vi "Build-timeline.vi"(8 "error in (no error)":errorcluster, 10 "Temp-timeline in":T1={"Previous point"={"Start time [µs]"=0, "End time [µs]"=0, "X [mm]"=0.0, "Y [mm]"=0.0, "Type"=enum."BeginJob", "Speed [mm/µs]"=0.0, "Direction [rad]"=0.0, "X [bit]"=0, "Y [bit]"=0, "Speed [bit/µs]"=0.0, "Power [W]"=0.0, "Power [bit]"=0, "JumpDelay"=0, "MarkDelay"=0, "PolyDelay"=0, "LaserOnDelay"=0, "LaserOffDelay"=0, "LaserPowerDelay"=0, "LaserEnableDelay"=0, "Xraw [mm]"=0.0, "Yraw [mm]"=0.0}, "Current point"={"Start time [µs]"=0, "End time [µs]"=0, "X [mm]"=0.0, "Y [mm]"=0.0, "Type"=enum."BeginJob", "Speed [mm/µs]"=0.0, "Direction [rad]"=0.0, "X [bit]"=0, "Y [bit]"=0, "Speed [bit/µs]"=0.0, "Power [W]"=0.0, "Power [bit]"=0, "JumpDelay"=0, "MarkDelay"=0, "PolyDelay"=0, "LaserOnDelay"=0, "LaserOffDelay"=0, "LaserPowerDelay"=0, "LaserEnableDelay"=0, "Xraw [mm]"=0.0, "Yraw [mm]"=0.0}, "Path"=[], "Current properties"={"ItemID"=0, "Start time"=0, "EffectiveOffset"=[0.0, 0.0], "EffectiveTranfsorm"=[[1.0, 0.0], [0.0, 1.0]], "Z-Offset"=0.0, "Units"=enum."mm", "LaserPower"=0, "Started"=FALSE, "Enabled"=FALSE, "FieldOffset"=[0.0, 0.0], "Offset"=[0.0, 0.0], "TransformEnable"=TRUE, "XYCalFactor"=196.0, "JumpSpeed"={"unit/us"=0.0, "Tick interval us"=0, "Bits per interval"=0}, "MarkSpeed"={"unit/us"=0.0, "Tick interval us"=0, "Bits per interval"=0}}}, 11 "JumpAbs in":refnum<class "JumpAbs.lvclass">) -> (0 "error out":errorcluster, 2 "Temp-timeline":T1={"Previous point"={"Start time [µs]"=0, "End time [µs]"=0, "X [mm]"=0.0, "Y [mm]"=0.0, "Type"=enum."BeginJob", "Speed [mm/µs]"=0.0, "Direction [rad]"=0.0, "X [bit]"=0, "Y [bit]"=0, "Speed [bit/µs]"=0.0, "Power [W]"=0.0, "Power [bit]"=0, "JumpDelay"=0, "MarkDelay"=0, "PolyDelay"=0, "LaserOnDelay"=0, "LaserOffDelay"=0, "LaserPowerDelay"=0, "LaserEnableDelay"=0, "Xraw [mm]"=0.0, "Yraw [mm]"=0.0}, "Current point"={"Start time [µs]"=0, "End time [µs]"=0, "X [mm]"=0.0, "Y [mm]"=0.0, "Type"=enum."BeginJob", "Speed [mm/µs]"=0.0, "Direction [rad]"=0.0, "X [bit]"=0, "Y [bit]"=0, "Speed [bit/µs]"=0.0, "Power [W]"=0.0, "Power [bit]"=0, "JumpDelay"=0, "MarkDelay"=0, "PolyDelay"=0, "LaserOnDelay"=0, "LaserOffDelay"=0, "LaserPowerDelay"=0, "LaserEnableDelay"=0, "Xraw [mm]"=0.0, "Yraw [mm]"=0.0}, "Path"=[], "Current properties"={"ItemID"=0, "Start time"=0, "EffectiveOffset"=[0.0, 0.0], "EffectiveTranfsorm"=[[1.0, 0.0], [0.0, 1.0]], "Z-Offset"=0.0, "Units"=enum."mm", "LaserPower"=0, "Started"=FALSE, "Enabled"=FALSE, "FieldOffset"=[0.0, 0.0], "Offset"=[0.0, 0.0], "TransformEnable"=TRUE, "XYCalFactor"=196.0, "JumpSpeed"={"unit/us"=0.0, "Tick interval us"=0, "Bits per interval"=0}, "MarkSpeed"={"unit/us"=0.0, "Tick interval us"=0, "Bits per interval"=0}}}, 3 "JumpAbs out":refnum<class "JumpAbs.lvclass">)   [LabVIEW 2013, in "HardwareCharacterization.lvlib" / "JumpAbs.lvclass"]
uses:
  JumpAbs.lvclass
  ScanParser/Path-buffer.ctl
  ScanParser/Point-buffer.ctl
  Elements.ctl
  ScanParser/Property-buffer.ctl
  ScanParser/Units.ctl
  ScanParser/Speed.ctl
  JumpAbs.lvclass/JumpAbs.ctl
  <vilib>/Analysis/baseanly.llb/A x Vector.vi
  <vilib>/Analysis/Matrix/Numeric/Conversions/Array To Matrix - RA2.vi
  <vilib>/Analysis/Matrix/NI_Matrix.lvlib
  <vilib>/Analysis/NI_AALBase.lvlib
  Element-XML.lvclass
  ScanParser/HC-ScanParser.lvclass
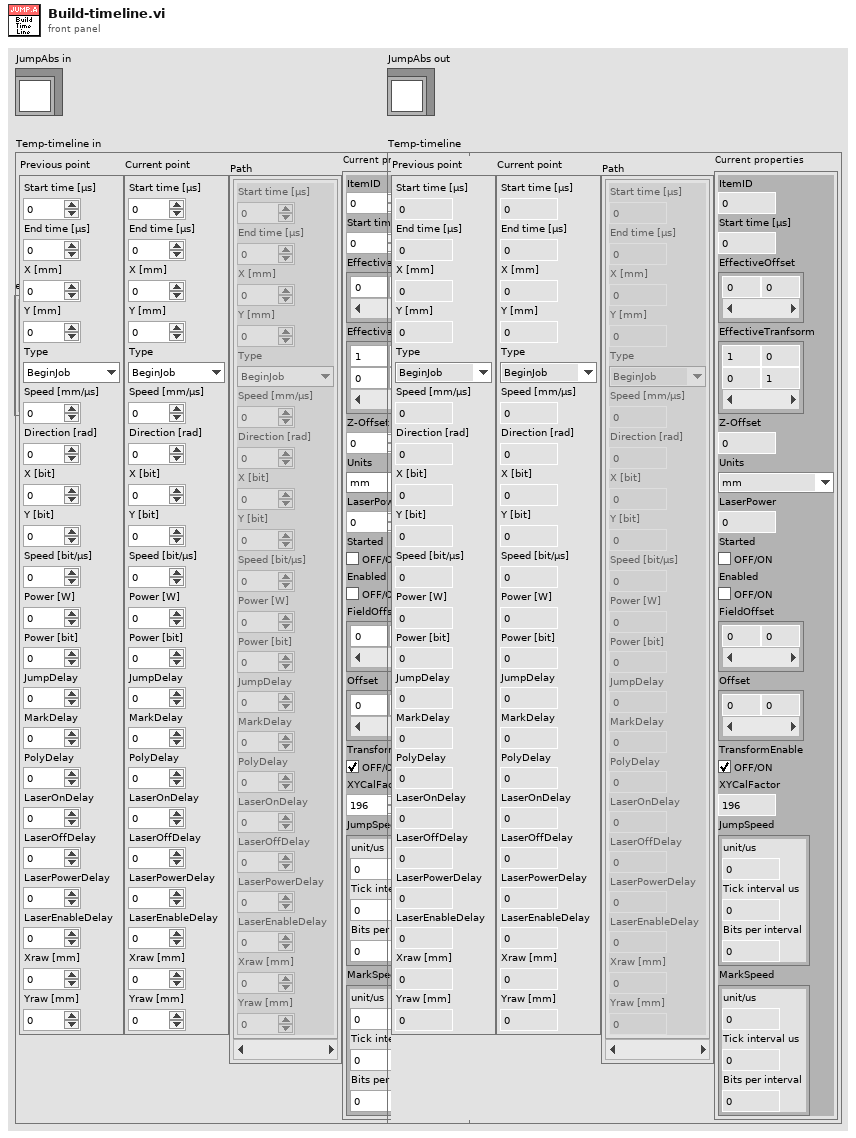
[diagram p1: front panel]
types:
  T1 = typedef "HardwareCharacterization.lvlib/HC-ScanParser.lvclass/Path-buffer.ctl" = cluster{"Previous point":T2, "Current point":T2, "Path":T2[], "Current properties":T4}
  T2 = typedef "HardwareCharacterization.lvlib/HC-ScanParser.lvclass/Point-buffer.ctl" = cluster{"Start time [µs]":i64, "End time [µs]":i64, "X [mm]":dbl, "Y [mm]":dbl, "Type":T3, "Speed [mm/µs]":dbl, "Direction [rad]":dbl, "X [bit]":i16, "Y [bit]":i16, "Speed [bit/µs]":dbl, "Power [W]":dbl, "Power [bit]":u8, "JumpDelay":i64, "MarkDelay":i64, "PolyDelay":i64, "LaserOnDelay":i64, "LaserOffDelay":i64, "LaserPowerDelay":i64, "LaserEnableDelay":i64, "Xraw [mm]":dbl, "Yraw [mm]":dbl}
  T3 = typedef "HardwareCharacterization.lvlib/Element-XML.lvclass/Elements.ctl" = enum16{"BeginJob", "WriteDigital", "WriteAnalog", "Set", "ApplicationEvent", "JumpAbs", "MarkAbs", "JumpRel", "MarkRel", "LongDelay", "EndJob"}
  T4 = typedef "HardwareCharacterization.lvlib/HC-ScanParser.lvclass/Property-buffer.ctl" = cluster{"ItemID":u32, "Start time":i64, "EffectiveOffset":dbl[], "EffectiveTranfsorm":dbl[][], "Z-Offset":sgl, "Units":T5, "LaserPower":u8, "Started":bool, "Enabled":bool, "FieldOffset":dbl[], "Offset":dbl[], "TransformEnable":bool, "XYCalFactor":dbl, "JumpSpeed":T6, "MarkSpeed":T6}
  T5 = typedef "HardwareCharacterization.lvlib/HC-ScanParser.lvclass/Units.ctl" = enum16{"bits", "mm", "inch", "mils"}
  T6 = typedef "HardwareCharacterization.lvlib/HC-ScanParser.lvclass/Speed.ctl" = cluster{"unit/us":dbl, "Tick interval us":u16, "Bits per interval":u16}
  T7 = typedef "NI_Matrix.lvlib/RealMatrix.ctl" = dbl[][]
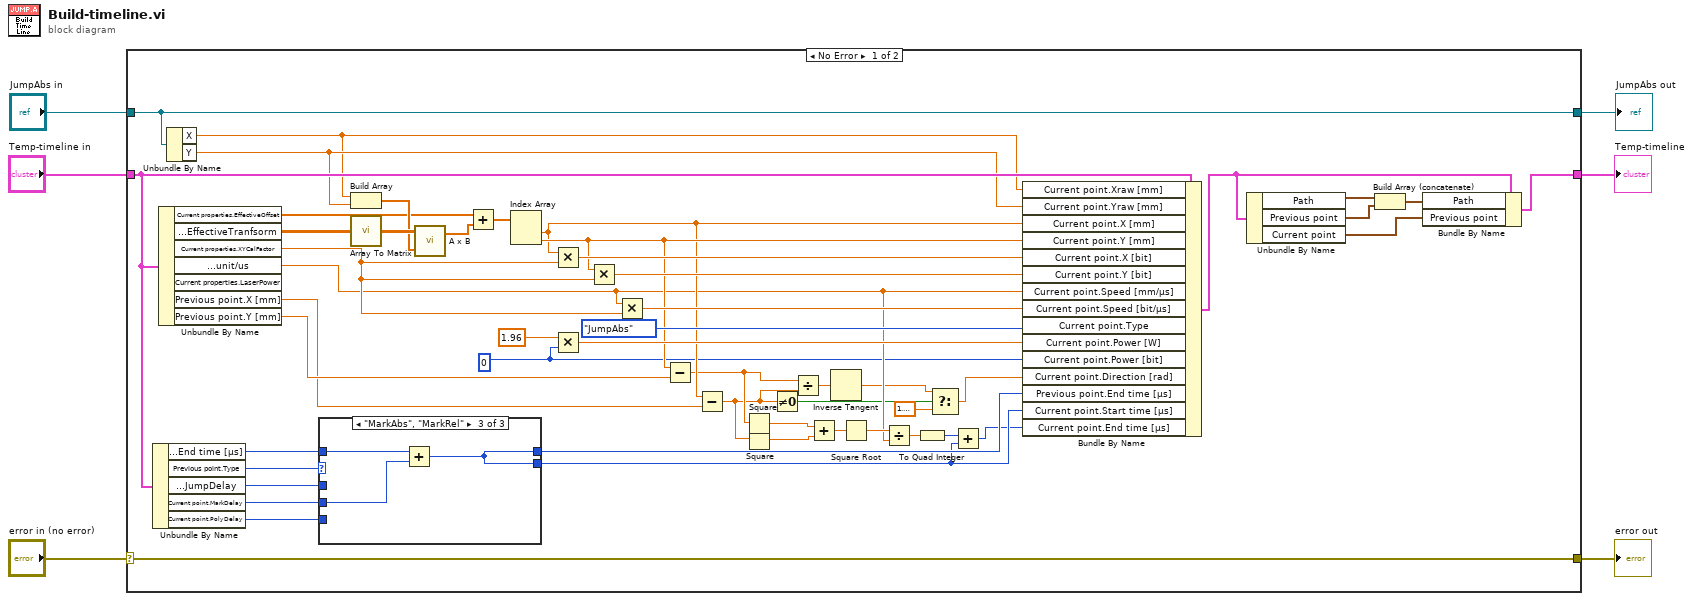
[diagram p0: block diagram]
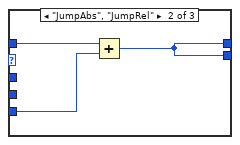
[diagram p3: hidden frame]
diagram:
  n1 = case shown="No Error" "error in (no error)" {
    selector: "error in (no error)" -> [w22 w67]
    tunnel: [w22 w67] -> w5
    tunnel: [w57 w66] -> w3
    tunnel: "JumpAbs in" -> [w57 w66]
    tunnel: "Temp-timeline in" -> [w39 w65]
    tunnel: [w20 w65] -> w1
    frame No Error {
      w15 = u8 0
      n2 = Unbundle By Name(w39) -> ("Previous point.End time [µs]"=w34:i64, "Previous point.Type"=w38:T3, "Current point.JumpDelay"=w37:i64, "Current point.MarkDelay"=w36:i64, "Current point.PolyDelay"=w35:i64)
      n3 = Unbundle By Name(w39) -> ("Current properties.EffectiveOffset"=w53:dbl[], "Current properties.EffectiveTranfsorm"=w56:dbl[][], "Current properties.XYCalFactor"=w47:dbl, "Current properties.JumpSpeed.unit/us"=w27:dbl, "Previous point.X [mm]"=w40:dbl, "Previous point.Y [mm]"=w42:dbl)  [unwired: 1 out]
      n4 = Unbundle By Name(w57) -> ("X"=w13:dbl, "Y"=w14:dbl)
      n5 = case shown="\"MarkAbs\", \"MarkRel\"" w38 {
        tunnel: w37 -> [_ _ _]
        tunnel: w36 -> [_ _ w62]
        tunnel: w35 -> [_ w60 _]
        tunnel: w34 -> [w58 w61 w64]
        tunnel: [w58 w59 w63] -> w33
        tunnel: [w58 w59 w63] -> w24
        frame "BeginJob", Default {
        }
        frame "JumpAbs", "JumpRel" {
          n6 = Add(x=w61, y=w60) -> (x+y=w59:i64)
        }
        frame "MarkAbs", "MarkRel" {
          n7 = Add(x=w64, y=w62) -> (x+y=w63:i64)
        }
      }
      n8 = Build Array(w13, w14) -> (w54:dbl[])
      n9 = call-poly <vilib>:"Array To Matrix.vi"("Real 2D Array"=w56) -> ("Real Matrix"=w55:T7)
      n10 = call-poly <vilib>:"A x B.vi"("Vector"=w54, "A"=w55) -> ("A x Vector"=w52:dbl[])  [unwired: 1 out]
      n11 = Add ("Add.vi")(x=w53, y=w52) -> (x+y=w51:dbl[])
      n12 = Index Array(array=w51) -> (element #1=w41:dbl, element #2=w43:dbl)  [unwired: 2 in]
      n13 = Multiply(x=w41, y=w47) -> (x*y=w50:dbl)
      n14 = Multiply(x=1.96, y=w15) -> (x*y=w45:dbl)
      n15 = Multiply(x=w43, y=w47) -> (x*y=w49:dbl)
      n16 = Multiply(x=w27, y=w47) -> (x*y=w48:dbl)
      n17 = Subtract(x=w43, y=w42) -> (x-y=w29:dbl)
      n18 = Subtract(x=w41, y=w40) -> (x-y=w12:dbl)
      n19 = Square(x=w29) -> (x^2=w32:dbl)
      n20 = Square(x=w12) -> (x^2=w31:dbl)
      n21 = Not Equal To 0?(x=w12) -> (x != 0?=w11:bool)
      n22 = Divide(x=w29, y=w12) -> (x/y=w10:dbl)
      n23 = Add(x=w32, y=w31) -> (x+y=w30:dbl)
      n24 = Inverse Tangent(1:w10) -> (0:w8:dbl)
      n25 = Square Root(x=w30) -> (sqrt(x)=w28:dbl)
      n26 = Divide(x=w28, y=w27) -> (x/y=w26:dbl)
      n27 = To Quad Integer(1:w26) -> (0:w25:i64)
      n28 = Select(t=w8, s=w11, f=1.5707963267948966) -> (s? t:f=w7:dbl)
      n29 = Add(x=w25, y=w24) -> (x+y=w23:i64)
      n30 = Bundle By Name(cluster=w39, "Current point.Xraw [mm]"=w13, "Current point.Yraw [mm]"=w14, "Current point.X [mm]"=w41, "Current point.Y [mm]"=w43, "Current point.X [bit]"=w50, "Current point.Y [bit]"=w49, "Current point.Speed [mm/µs]"=w27, "Current point.Speed [bit/µs]"=w48, "Current point.Type"=Elements."JumpAbs", "Current point.Power [W]"=w45, "Current point.Power [bit]"=w15, "Current point.Direction [rad]"=w7, "Previous point.End time [µs]"=w33, "Current point.Start time [µs]"=w24, "Current point.End time [µs]"=w23) -> (w21:T1)
      n31 = Unbundle By Name(w21) -> ("Path"=w19:T2[], "Previous point"=w18:T2, "Current point"=w16:T2)
      n32 = Build Array (concatenate)(w19, w18) -> (w17:T2[])
      n33 = Bundle By Name(cluster=w21, "Path"=w17, "Previous point"=w16) -> (w20:T1)
    }
    frame Error {
    }
  }
  "error out" <- w5
  "JumpAbs out" <- w3
  "Temp-timeline" <- w1
